vi "Connect.vi"(8 "error in (no error)":errorcluster, 11 "SolarSystems M266 in":refnum<class "SolarSystems M266.lvclass">) -> (0 "error out":errorcluster, 3 "SolarSystems M266 out":refnum<class "SolarSystems M266.lvclass">)   [LabVIEW 2014, in "SolarSystems M266.lvclass"]
uses:
  SolarSystems M266.lvclass
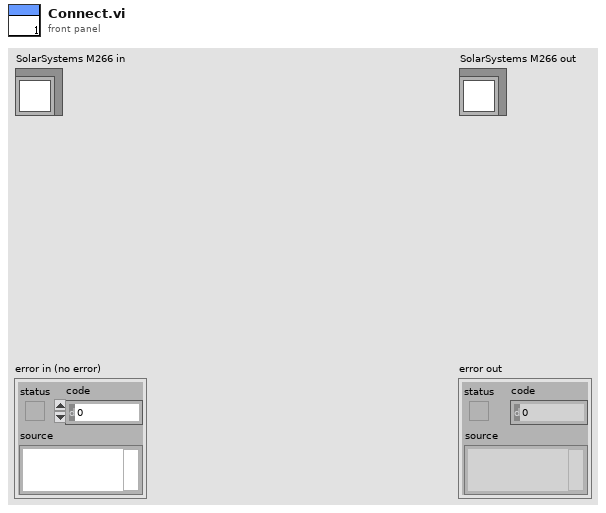
[diagram p1: front panel]
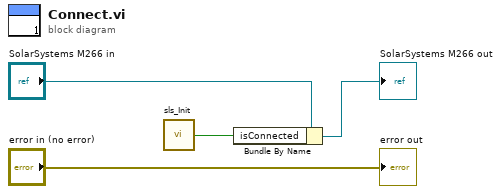
[diagram p0: block diagram]
diagram:
  n1 = call "sls_Init.vi"() -> ("Result"=w3:bool)  [unwired: 1 in]
  n2 = Bundle By Name(cluster="SolarSystems M266 in", "isConnected"=w3) -> (→"SolarSystems M266 out":refnum<class "SolarSystems M266.lvclass">)
  "error out" <- "error in (no error)"
